vi "UI-XListGraph-Example.vi"() -> ()   [LabVIEW 2017]
uses:
  XListGraph.xctl
  <userlib>/_OpenG.lib/numeric/numeric.llb/Random Number Within Range - DBL__ogtk.vi
  <vilib>/measure/maspectr.llb/FFT Power Spectrum for 1 Chan.vi
  <vilib>/measure/NI_MABase.lvlib
  <vilib>/measure/NI_MAPro.lvlib
panel:
  out "XGraph":waveform(dbl)[](xcontrol)
  out "fft":waveform(dbl)[](xcontrol)
  in  "Visible":bool
  in  "Set List Window Visible":bool
  in  "Select Sine":bool
  in  "Hide Sine":bool
  in  "Show Sine":bool
  out "Plot Names":string[](array[string])
  out "Visible Plot Names":string[](array[string])
  out "Selected Plot Names":string[](array[string])
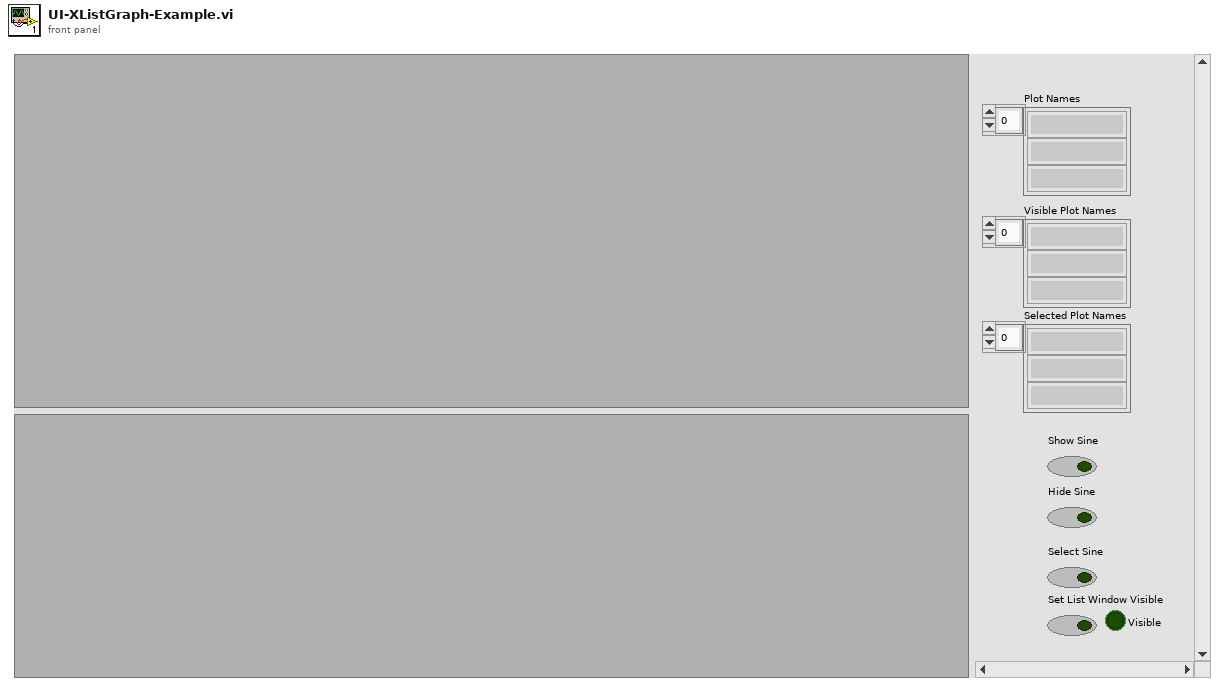
[diagram p1: front panel]
types:
  T1 = typedef "XListGraph.lvlib/XListGraph.xctl/def-XListGraphOper.ctl" = u16
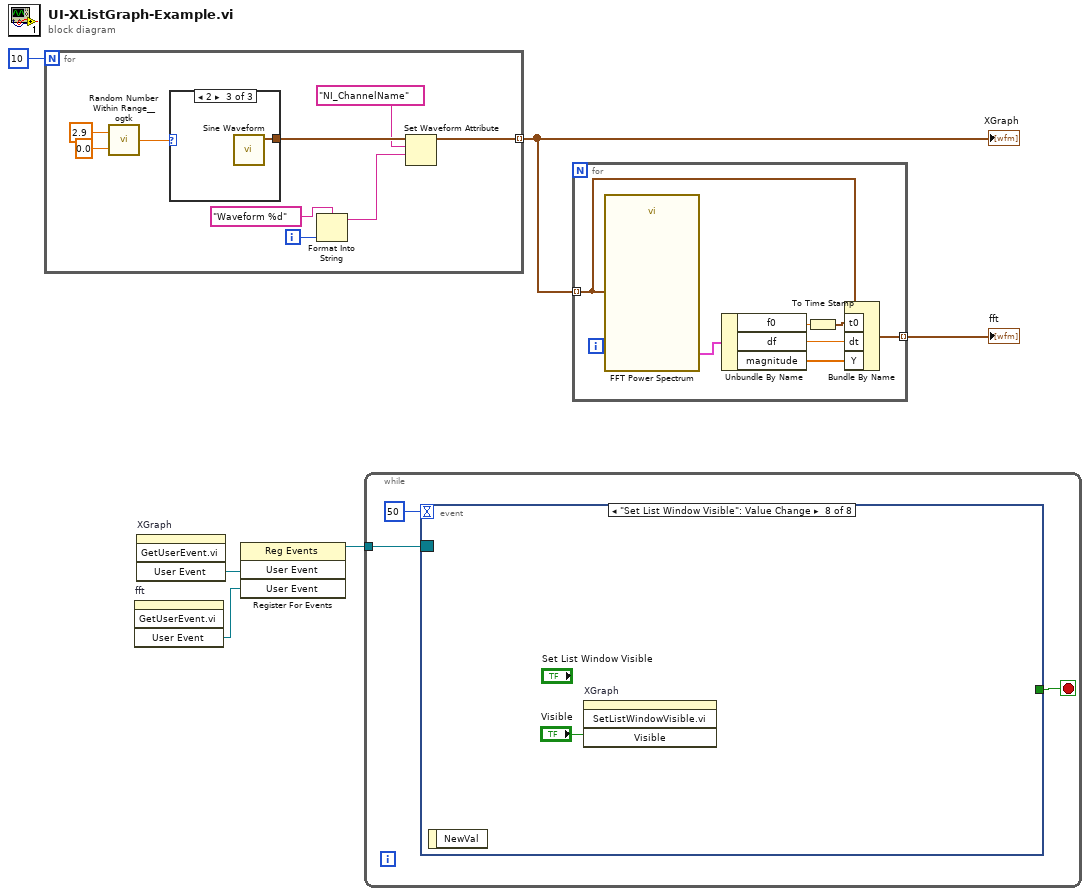
[diagram p0: block diagram]
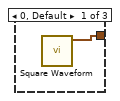
[diagram p2: hidden frame]
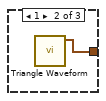
[diagram p3: hidden frame]
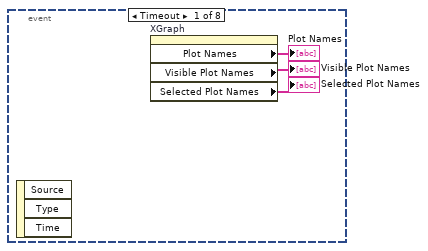
[diagram p4: hidden frame]
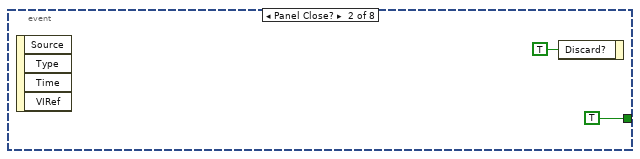
[diagram p5: hidden frame]
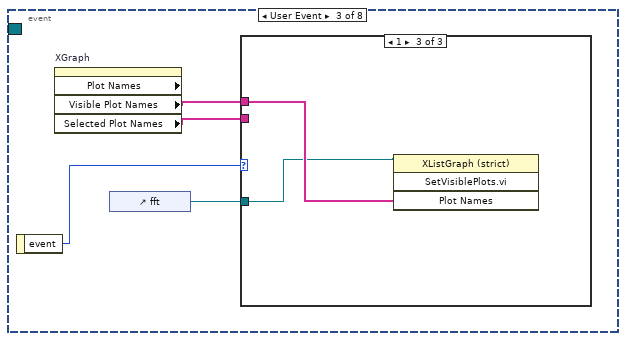
[diagram p6: hidden frame]
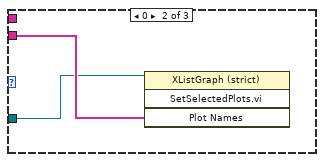
[diagram p8: hidden frame]
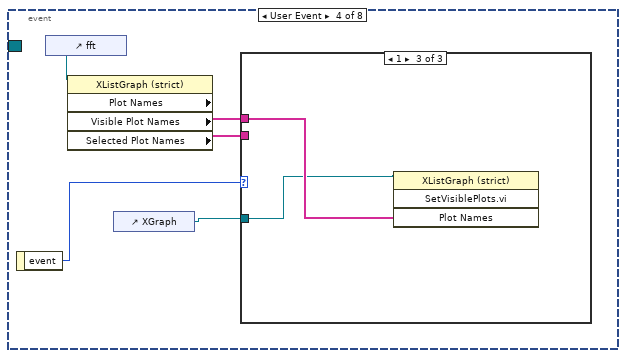
[diagram p9: hidden frame]
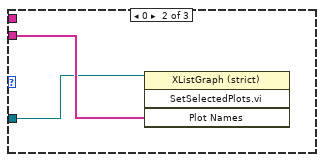
[diagram p11: hidden frame]
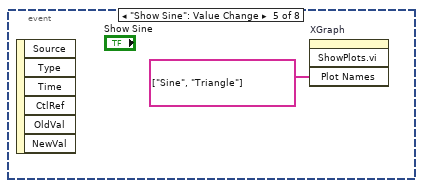
[diagram p12: hidden frame]
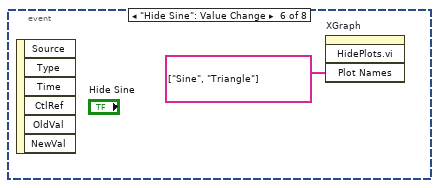
[diagram p13: hidden frame]
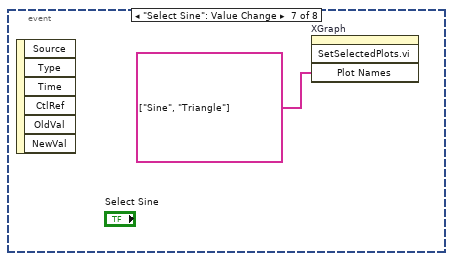
[diagram p14: hidden frame]
diagram:
  n1 = for {
    N: 10 -> [_]
    tunnel: [w14] -> w4 mode=indexing
    i -> [w9]
    n2 = call-poly <userlib>:"Random Number Within Range__ogtk.vi"("High"=2.9, "Low"=0.0) -> ("Random Number"=w13:dbl)  [unwired: 3 in]
    n3 = case shown="2" w13 {
      tunnel: [w16 w17 w18] -> w15
      frame 0, Default {
        n4 = call <vilib>:"Square Waveform.vi"() -> ("signal out"=w16:waveform(dbl))  [unwired: 10 in, 1 out]
      }
      frame 1 {
        n5 = call <vilib>:"Triangle Waveform.vi"() -> ("signal out"=w17:waveform(dbl))  [unwired: 10 in, 1 out]
      }
      frame 2 {
        n6 = call <vilib>:"Sine Waveform.vi"() -> ("signal out"=w18:waveform(dbl))  [unwired: 10 in, 1 out]
      }
    }
    n7 = Format Into String(format string="Waveform %d", w9) -> (resulting string=w10:string)  [unwired: 2 in, 1 out]
    n8 = Set Waveform Attribute(5:w10, 6:"NI_ChannelName" ("name"), 7:w15) -> (3:w14:waveform(dbl))  [unwired: 1 in, 2 out]
  }
  "XGraph" <- w4
  n9 = invoke on="fft" class="XListGraph (strict)" method="GetUserEvent.vi"() -> ("User Event"=w2:refnum<user-event>)  [unwired: 4 in, 3 out]
  n10 = invoke on="XGraph" class="XListGraph (strict)" method="GetUserEvent.vi"() -> ("User Event"=w5:refnum<user-event>)  [unwired: 4 in, 3 out]
  n11 = register-events(w5, w2) -> (reference out=w6:refnum<event-registration>)  [unwired: 2 in, 1 out]
  n12 = while {
    tunnel: w6 -> [w19]
    stop <- w20 stop-if-true
    n13 = event shown="[7] \"Set List Window Visible\": Value Change" {
      selector: w19 -> [_ _ _ _ _ _ _ _]
      dyn-events: _ -> [_ _ _ _ _ _ _ _]
      timeout: 50 -> [_ _ _ _ _ _ _ _]
      tunnel: [_ TRUE _ _ _ _ _ _] -> w20
      event Timeout {
        n14 = event-data() -> ()  [unwired: 1 in, 3 out]
        n15 = property on="XGraph" class="XListGraph (strict)"() -> ("Plot Names"=→"Plot Names":string[], "Visible Plot Names"=→"Visible Plot Names":string[], "Selected Plot Names"=→"Selected Plot Names":string[])  [unwired: 2 in, 2 out]
      }
      event Panel Close? {
        n16 = event-data() -> ()  [unwired: 1 in, 4 out]
        n17 = event-data("Discard?"=TRUE) -> ()  [unwired: 1 in, 1 out]
      }
      event User Event {
        n18 = event-data() -> ("event"=w30:T1)  [unwired: 1 in]
        n19 = property on="XGraph" class="XListGraph (strict)" props=["Plot Names", "Visible Plot Names", "Selected Plot Names"]() -> ("Visible Plot Names"=w28:string[], "Selected Plot Names"=w29:string[])  [unwired: 2 in, 3 out]
        n20 = control-ref of="fft"() -> (w27:refnum<vi>)
        n21 = case shown="1" w30 {
          tunnel: w29 -> [_ w32 _]
          tunnel: w28 -> [_ _ w34]
          tunnel: w27 -> [_ w31 w33]
          frame Default {
          }
          frame 0 {
            n22 = invoke on="Invoke Node" class="XListGraph (strict)" method="SetSelectedPlots.vi"(reference=w31, "Plot Names"=w32) -> ()  [unwired: 2 in, 4 out]
          }
          frame 1 {
            n23 = invoke on="Invoke Node" class="XListGraph (strict)" method="SetVisiblePlots.vi"(reference=w33, "Plot Names"=w34) -> ()  [unwired: 2 in, 4 out]
          }
        }
      }
      event User Event {
        n24 = event-data() -> ("event"=w39:T1)  [unwired: 1 in]
        n25 = control-ref of="fft"() -> (w36:refnum<vi>)
        n26 = property on="Property Node" class="XListGraph (strict)" props=["Plot Names", "Visible Plot Names", "Selected Plot Names"](reference=w36) -> ("Visible Plot Names"=w37:string[], "Selected Plot Names"=w38:string[])  [unwired: 1 in, 3 out]
        n27 = control-ref of="XGraph"() -> (w35:refnum<vi>)
        n28 = case shown="1" w39 {
          tunnel: w38 -> [_ w41 _]
          tunnel: w37 -> [_ _ w43]
          tunnel: w35 -> [_ w40 w42]
          frame Default {
          }
          frame 0 {
            n29 = invoke on="Invoke Node" class="XListGraph (strict)" method="SetSelectedPlots.vi"(reference=w40, "Plot Names"=w41) -> ()  [unwired: 2 in, 4 out]
          }
          frame 1 {
            n30 = invoke on="Invoke Node" class="XListGraph (strict)" method="SetVisiblePlots.vi"(reference=w42, "Plot Names"=w43) -> ()  [unwired: 2 in, 4 out]
          }
        }
      }
      event "Show Sine": Value Change {
        n31 = event-data() -> ()  [unwired: 1 in, 6 out]
        n32 = invoke on="XGraph" class="XListGraph (strict)" method="ShowPlots.vi"("Plot Names"=string[] ["Sine", "Triangle"]) -> ()  [unwired: 3 in, 4 out]
      }
      event "Hide Sine": Value Change {
        n33 = event-data() -> ()  [unwired: 1 in, 6 out]
        n34 = invoke on="XGraph" class="XListGraph (strict)" method="HidePlots.vi"("Plot Names"=string[] ["Sine", "Triangle"]) -> ()  [unwired: 3 in, 4 out]
      }
      event "Select Sine": Value Change {
        n35 = event-data() -> ()  [unwired: 1 in, 6 out]
        n36 = invoke on="XGraph" class="XListGraph (strict)" method="SetSelectedPlots.vi"("Plot Names"=string[] ["Sine", "Triangle"]) -> ()  [unwired: 3 in, 4 out]
      }
      event "Set List Window Visible": Value Change {
        n37 = event-data() -> ()  [unwired: 1 in, 1 out]
        n38 = invoke on="XGraph" class="XListGraph (strict)" method="SetListWindowVisible.vi"("Visible"="Visible") -> ()  [unwired: 3 in, 4 out]
      }
    }
  }
  n39 = for {
    tunnel: w4 -> [w48] mode=indexing
    tunnel: [w49] -> w3 mode=indexing
    n40 = call-poly <vilib>:"FFT Power Spectrum.vi"("time signal"=w48) -> ("power spectrum"=w54:cluster{"f0":dbl, "df":dbl, "magnitude":dbl[]})  [unwired: 7 in, 3 out]
    n41 = Unbundle By Name(w54) -> ("f0"=w53:dbl, "df"=w52:dbl, "magnitude"=w51:dbl[])
    n42 = To Time Stamp(1:w53) -> (0:w50:timestamp)
    n43 = Bundle By Name(cluster=w48, "t0"=w50, "dt"=w52, "Y"=w51) -> (w49:waveform(dbl))
  }
  "fft" <- w3
